vi "UMLEditor_GetActiveWindow.vi"(8 "error in (no error)":errorcluster) -> (0 "error out":errorcluster, 1 "Project Explorer":bool, 2 "Active Window":string)   [LabVIEW 2016]
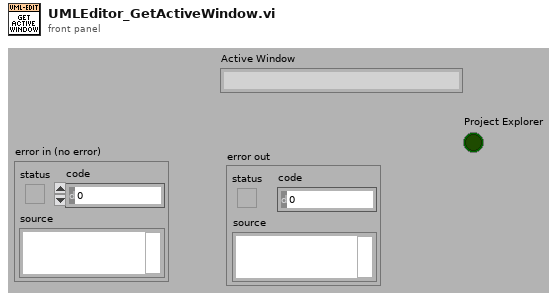
[diagram p1: front panel]
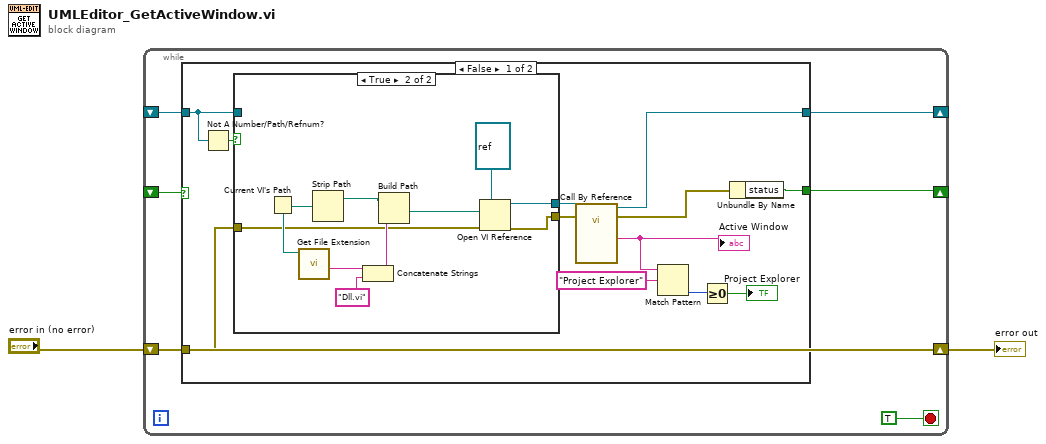
[diagram p0: block diagram]
diagram:
  n1 = while {
    shift-right: [w7] -> _
    shift-left: _ -> [w8]
    shift-right: [w5] -> w2
    shift-left: "error in (no error)" -> [w5]
    shift-right: [w4] -> _
    shift-left: _ -> [w3]
    stop <- TRUE stop-if-true
    n2 = case shown="False" w3 {
      selector: w3 -> [_ w34]
      tunnel: w8 -> [w13 w33]
      tunnel: [w17 w33] -> w7
      tunnel: w5 -> [w16 _]
      tunnel: [w14 w34] -> w4
      frame False {
        n3 = Not A Number/Path/Refnum?(number/path/refnum=w13) -> (NaN/Path/Refnum?=w18:bool)
        n4 = case shown="True" w18 {
          tunnel: [w22 w26] -> w20
          tunnel: [w21 w25] -> w19
          tunnel: w13 -> [w22 _]
          tunnel: w16 -> [w21 w24]
          frame False {
          }
          frame True {
            n5 = Current VI's Path() -> (path=w31:path)
            n6 = call <vilib>:"Get File Extension.vi"("file"=w31) -> ("filename without extension"=w23:string)  [unwired: 1 in, 9 out]
            n7 = Strip Path(path=w31) -> (stripped path=w29:path)  [unwired: 1 out]
            n8 = Concatenate Strings(w23, "Dll.vi" ("format string")) -> (w28:string)
            n9 = Build Path(base path=w29, name or relative path=w28) -> (appended path=w27:path)
            n10 = Open VI Reference(type specifier VI Refnum (for type only)=refnum<vi> refnum, vi path=w27, error in (no error)=w24) -> (vi reference=w26:refnum<vi>, error out=w25:errorcluster)  [unwired: 3 out]
          }
        }
        n11 = call-by-ref "?"(reference=w20, error in=w19) -> (reference out=w17:refnum<vi>, error out=w15:errorcluster, "Active Window"=w12:string)  [unwired: 11 in]
        "Active Window" <- w12
        n12 = Match Pattern(string=w12, regular expression="Project Explorer") -> (offset past match=w10:i32)  [unwired: 4 out]
        n13 = Greater Or Equal To 0?(x=w10) -> (x >= 0?=→"Project Explorer":bool)
        n14 = Unbundle By Name(w15) -> ("status"=w14:bool)
      }
      frame True {
      }
    }
  }
  "error out" <- w2
